vi "StartStop.vi"(10 "STOP":bool, 11 "START":bool) -> ()   [LabVIEW 2017]
uses:
  Program Files/National Instruments/LabVIEW 2019/user.lib/HapticSTM/HapticSTM.lvlib
panel:
  in  "CALIBRATE":bool
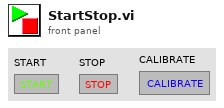
[diagram p1: front panel]
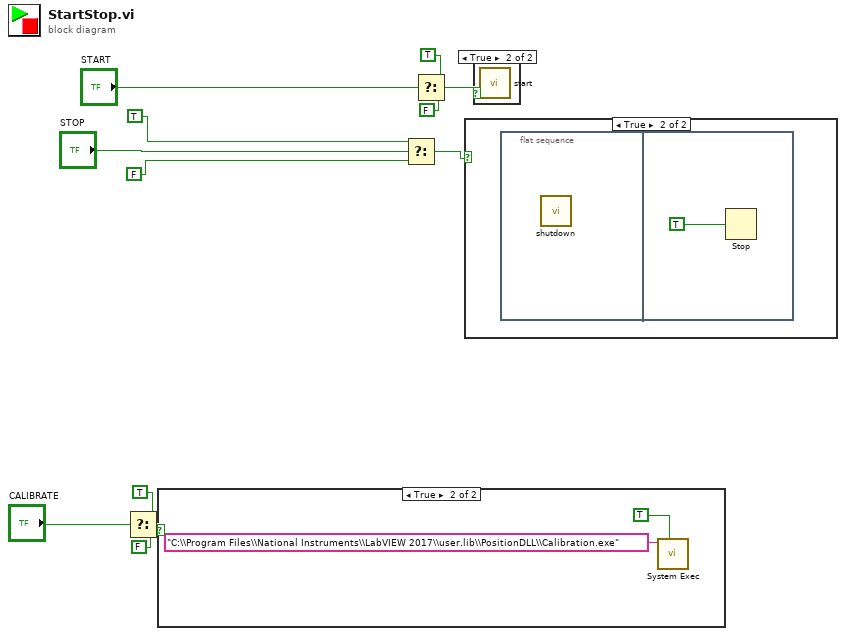
[diagram p0: block diagram]
diagram:
  n1 = Select(t=TRUE, s="CALIBRATE", f=FALSE) -> (s? t:f=w2:bool)
  n2 = case shown="True" w2 {
    frame False {
    }
    frame True {
      n3 = call <vilib>:"System Exec.vi"("wait until completion? (T)"=TRUE, "command line"="C:\\Program Files\\National Instruments\\LabVIEW 2017\\user.lib\\PositionDLL\\Calibration.exe") -> ()  [unwired: 6 in, 4 out]
    }
  }
  n4 = Select(t=TRUE, s="STOP", f=FALSE) -> (s? t:f=w9:bool)
  n5 = Select(t=TRUE, s="START", f=FALSE) -> (s? t:f=w5:bool)
  n6 = case shown="True" w9 {
    frame False {
    }
    frame True {
      n7 = flat-sequence {
        frame #0 {
          n8 = call "shutdown.vi"() -> ()  [unwired: 12 in]
        }
        frame #1 {
          n9 = Stop(stop? (T)=TRUE) -> ()
        }
      }
    }
  }
  n10 = case shown="True" w5 {
    frame False {
    }
    frame True {
      n11 = call "start.vi"() -> ()  [unwired: 11 in, 1 out]
    }
  }
